vi "Set Steering Frame.vi"(8 "error in (no error)":errorcluster, 9 "differential frame velocity":dbl[](array[numeric])=[0.0, 0.0, 0.0], 10 "mecanum frame velocity":dbl[](array[numeric])=[0.0, 0.0, 0.0], 11 "Steering Frame in":T3) -> (0 "error out":errorcluster, 3 "Steering Frame out":T3)   [LabVIEW 2012]
uses:
  <vilib>/robotics/Steering/Class Type Definitions/Mecanum Steering Frame.ctl
  <vilib>/robotics/Steering/Mecanum Steering Frame/NI_Robotics_Mecanum Steering Frame.lvclass
  <vilib>/robotics/Steering/Class Type Definitions/Differential Steering Frame.ctl
  <vilib>/robotics/Steering/Differential Steering Frame/NI_Robotics_Differential Steering Frame.lvclass
  <vilib>/robotics/Steering/Steering Frame/Apply Steering Frame Velocity to Wheels.vi
  <vilib>/robotics/Steering/Steering Frame/NI_Robotics_Steering Frame.lvclass
  <vilib>/robotics/Steering/Class Type Definitions/NI_Robotics_Steering Class Types.lvlib
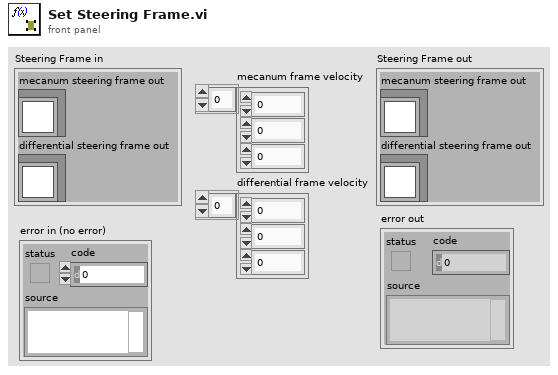
[diagram p1: front panel]
types:
  T1 = typedef "NI_Robotics_Steering Class Types.lvlib/Mecanum Steering Frame.ctl" = refnum<class "NI_Robotics_Mecanum Steering Frame.lvclass">
  T2 = typedef "NI_Robotics_Steering Class Types.lvlib/Differential Steering Frame.ctl" = refnum<class "NI_Robotics_Differential Steering Frame.lvclass">
  T3 = cluster{"mecanum steering frame out":T1, "differential steering frame out":T2}
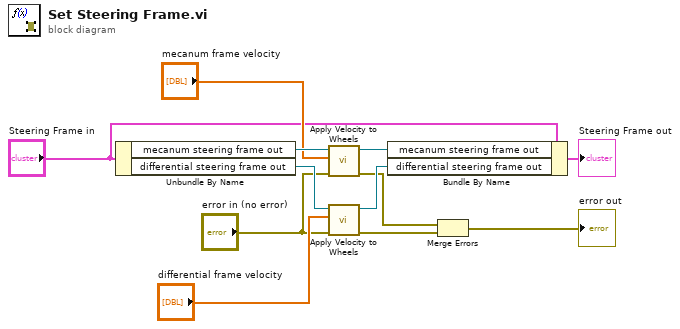
[diagram p0: block diagram]
diagram:
  n1 = Unbundle By Name("Steering Frame in") -> ("mecanum steering frame out"=w12:T1, "differential steering frame out"=w11:T2)
  n2 = call-poly <vilib>:"Apply Velocity to Wheels.vi"("error in (no error)"="error in (no error)", "steering frame velocity"="mecanum frame velocity", "steering frame in"=w12) -> ("error out"=w3:errorcluster, "steering frame out"=w10:T1)  [unwired: 5 in, 2 out]
  n3 = call-poly <vilib>:"Apply Velocity to Wheels.vi"("error in (no error)"="error in (no error)", "steering frame velocity"="differential frame velocity", "steering frame in"=w11) -> ("error out"=w2:errorcluster, "steering frame out"=w9:T2)  [unwired: 5 in, 2 out]
  n4 = Bundle By Name(cluster="Steering Frame in", "mecanum steering frame out"=w10, "differential steering frame out"=w9) -> (→"Steering Frame out":T3)
  n5 = Merge Errors(w3, w2) -> (→"error out":errorcluster)
